vi "Sensor Read.vi"   [LabVIEW 2016]
uses:
  Drive/Drive Globals.vi
  Rotation/Rotation Globals.vi
types:
  T1 = typedef "CTRE_PigeonIMU_DeviceRef.ctl" = cluster{"DeviceStatus":errorcluster, "Device Number":u8, "Type":T2, "Device ID":u32}
  T2 = typedef "CTRE_PigeonIMU_ConnectionType.ctl" = u32
  T3 = typedef "CTRE_PigeonIMU_GlobalStatus.ctl" = cluster{"PigeonState":T4, "FusedHeading":cluster{"Heading":dbl, "Valid?":bool, "Fusing?":bool}, "YPR":cluster{"Yaw":dbl, "Pitch":dbl, "Roll":dbl}, "Compass":cluster{"Heading":dbl, "Magnitude":dbl, "Absolute Heading":dbl}, "Accelerometer":cluster{"Biased":cluster{"X":i16, "Y":i16, "Z":i16, "Norm":i16}, "Angles":cluster{"XZ Tilt":dbl, "YZ Tilt":dbl, "XY Tilt":dbl}}, "Magnetometer":cluster{"Raw":cluster{"X":i16, "Y":i16, "Z":i16}, "Biased":cluster{"X":i16, "Y":i16, "Z":i16}}, "Gyro":cluster{"X":dbl, "Y":dbl, "Z":dbl, "Norm":dbl}, "6D Quaternian":cluster{"W":dbl, "X":dbl, "Y":dbl, "Z":dbl}, "Temp. (C)":dbl, "UpTime":u32, "StartupStatus":cluster{"ResetCount":i32, "ResetFlags":i32, "FirmwareVersion":i32, "HasReset?":bool}, "Calibration":cluster{"CurrentMode":T5, "LastCalError":i32, "CalBooting?":bool}, "CAN Error":errorcluster, "AccumGyro":cluster{"X":dbl, "Y":dbl, "Z":dbl}, "Usage Frame":u32}
  T4 = typedef "CTRE_PigeonIMU_PigeonState.ctl" = enum16{"NoComm", "Initializing", "Ready", "UserCalibration"}
  T5 = typedef "CTRE_PigeonIMU_CalibrationMode.ctl" = u16
  T6 = typedef "WPI_SwitchDevRef.ctl" = cluster{"DevStatus":errorcluster, "DIO Channel":T7, "CntIndex":T8, "Normally Closed":bool}
  T7 = typedef "FPGA_DIOChannel.ctl" = enum8{"DIO 0", "DIO 1", "DIO 2", "DIO 3", "DIO 4", "DIO 5", "DIO 6", "DIO 7", "DIO 8", "DIO 9", "DIO MXP 0", "DIO MXP 1", "DIO MXP 2", "DIO MXP 3", "DIO MXP 4", "DIO MXP 5", "DIO MXP 6", "DIO MXP 7", "DIO MXP 8", "DIO MXP 9", "DIO MXP 10", "DIO MXP 11", "DIO MXP 12", "DIO MXP 13", "DIO MXP 14", "DIO MXP 15", "SPI Port CS1", "SPI Port CS2", "SPI Port CS3", "SPI Port MISO", "SPI Port MOSI", "Invalid"}
  T8 = typedef "FPGA_CounterCtrSystemIndex.ctl" = enum8{"Ctr 0", "Ctr 1", "Ctr 2", "Ctr 3", "Ctr 4", "Ctr 5", "Ctr 6", "Ctr 7", "Invalid"}
  T9 = typedef "WPI_EncoderDevRef.ctl" = cluster{"DevStatus":errorcluster, "EncoderIndex":T10, "CounterIndex":T8, "DistancePerCount":dbl, "Decoding Type":T11}
  T10 = typedef "FPGA_EncoderIdx.ctl" = enum8{"Enc 0", "Enc 1", "Enc 2", "Enc 3", "Enc 4", "Enc 5", "Enc 6", "Enc 7", "Invalid"}
  T11 = typedef "WPI_EncoderType.ctl" = enum16{"1x", "2x", "4x"}
  T12 = typedef "WPI_MotorControlDeviceRef.ctl" = cluster{"DeviceStatus":errorcluster, "Type":T13, "PWM":cluster{"PWM Channel":T14, "DeadBand":T15}, "CAN":cluster{"Device Number":u8, "SetOutput VI Ref":variant, "GetOutput VI Ref":variant, "Enable VI Ref":variant, "Disable VI Ref":variant, "Data":variant}, "Invert":bool}
  T13 = typedef "WPI_MotorControlType.ctl" = enum16{"PWM", "CAN"}
  T14 = typedef "FPGA_DIOPWMChannel.ctl" = enum8{"PWM 0", "PWM 1", "PWM 2", "PWM 3", "PWM 4", "PWM 5", "PWM 6", "PWM 7", "PWM 8", "PWM 9", "PWM MXP 0", "PWM MXP 1", "PWM MXP 2", "PWM MXP 3", "PWM MXP 4", "PWM MXP 5", "PWM MXP 6", "PWM MXP 7", "PWM MXP 8", "PWM MXP 9", "Invalid"}
  T15 = typedef "WPI_PWMDeadband.ctl" = cluster{"Name":string, "maxPositivePwm":i32, "minPositivePwm":i32, "centerPwm":i32, "maxNegativePwm":i32, "minNegativePwm":i32, "angularRange":u16}
  T16 = typedef "WPI_CANTalonSRX_GlobalStatus.ctl" = cluster{"Applied Throttle":dbl, "Module Enabled":bool, "CAN Error":errorcluster, "Closed Loop Error":dbl, "Forward Limit Switch Closed":bool, "Reverse Limit Switch Closed":bool, "Sensor Position":dbl, "Sensor Velocity":dbl, "Current":dbl, "Sticky Fault - Over Temp":bool, "Sticky Fault - Under Voltage":bool, "Sticky Fault - Forward Limit":bool, "Sticky Fault - Reverse Limit":bool, "Sticky Fault - Forward Soft Limit":bool, "Sticky Fault - Reverse Soft Limit":bool, "Brake is Enabled":bool, "Encoder Position":dbl, "Encoder Velocity":dbl, "Encoder Index Count":dbl, "Encoder A Pin State":bool, "Encoder B Pin State":bool, "Encoder Index Pin State":bool, "Analog In":dbl, "Analog In Velocity":dbl, "Temperature (C)":dbl, "Battery Voltage":dbl, "Control 5 Is Supported":bool, "Current Profile Slot Select":dbl, "Pos Div 8":bool, "Vel Div 4":bool, "Pulse Width Position":i32, "Pulse Width Velocity":i32, "Pulse Width Rise To Rise (us)":i32, "Pulse Width Rise To Fall (us)":i32, "Mot Prof Active Is Under Run":bool, "Mot Prof Active Has Under Run":bool, "Mot Prof Active Is Last":bool, "Mot Prof Active Velocity Only":bool, "Mot Prof Active Is Valid":bool, "Mot Prof Buffer Is Full":bool, "Mot Prof Active Profile Slot Select":i32, "Mot Prof NextID":i32, "Mot Prof Count":i32, "Mot Prof Active Velocity":dbl, "Mot Prof Active Position":dbl, "Mot Prof Output Enable":i32, "UsageFrame":u32, "Motion Magic Active Trajectory":cluster{"Velocity":dbl, "Position":dbl}}
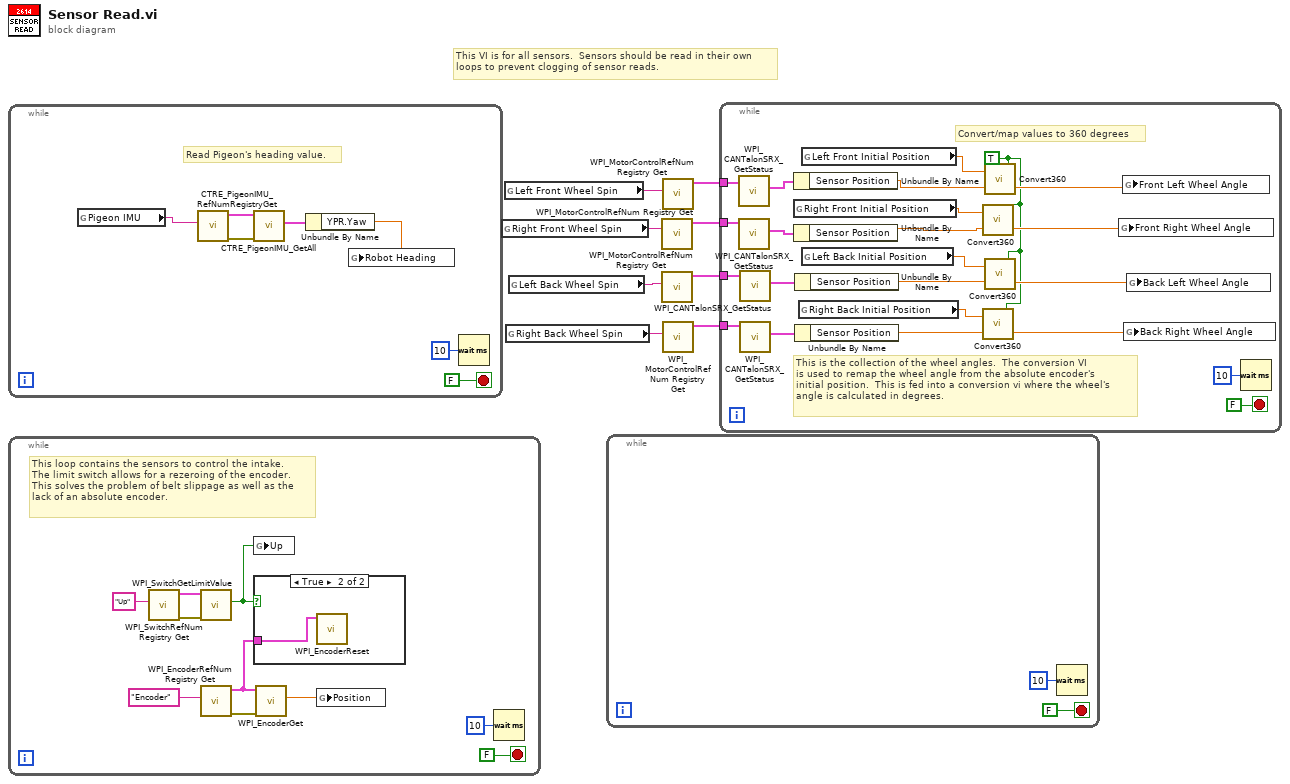
[diagram p0: block diagram]
diagram:
  # "This VI is for all sensors.  Sensors should be read in their own \nloops to prevent clogging of sensor reads."
  n1 = while {
    stop <- FALSE stop-if-true
    # "Read Pigeon's heading value."
    n2 = global read "Drive Globals.vi" "Pigeon IMU"() -> (w13:string)
    n3 = call <vilib>:"CTRE_PigeonIMU_RefNumRegistryGet.vi"("refnum name"=w13) -> ("error out"=w12:errorcluster, "PigeonIMUDevRef"=w11:T1)  [unwired: 9 in]
    n4 = call <vilib>:"CTRE_PigeonIMU_GetAll.vi"("error in (no error)"=w12, "PigeonIMUDevRef"=w11) -> ("Get All"=w10:T3)  [unwired: 7 in, 2 out]
    n5 = Unbundle By Name(w10) -> ("YPR.Yaw"=w9:dbl)
    n6 = global write "Drive Globals.vi" "Robot Heading"(w9) -> ()
    n7 = Wait (ms)(milliseconds to wait=u32 10) -> ()  [unwired: 1 out]
  }
  n8 = while {
    stop <- FALSE stop-if-true
    # "This loop contains the sensors to control the intake. \nThe limit switch allows for a rezeroing of the encoder.\nThis solves the problem of belt slippage as well as the\nlack of an absolute encoder."
    n9 = call <vilib>:"WPI_SwitchRefNum Registry Get.vi"("refnum name"="Up") -> ("error out"=w20:errorcluster, "SwitchDevRef"=w19:T6)  [unwired: 9 in]
    n10 = call <vilib>:"WPI_SwitchGetLimitValue.vi"("error in (no error)"=w20, "SwitchDevRef"=w19) -> ("Switch Pressed"=w17:bool)  [unwired: 7 in, 2 out]
    n11 = call <vilib>:"WPI_EncoderRefNum Registry Get.vi"("refnum name"="Encoder") -> ("error out"=w22:errorcluster, "EncoderDevRef"=w16:T9)  [unwired: 9 in]
    n12 = global write "Rotation Globals.vi" "Up"(w17) -> ()
    n13 = case shown="True" w17 {
      tunnel: w16 -> [_ w26]
      frame False {
      }
      frame True {
        n14 = call <vilib>:"WPI_EncoderReset.vi"("EncoderDevRef"=w26) -> ()  [unwired: 9 in, 2 out]
      }
    }
    n15 = call <vilib>:"WPI_EncoderGet.vi"("error in (no error)"=w22, "EncoderDevRef"=w16) -> ("Distance"=w21:dbl)  [unwired: 4 in, 5 out]
    n16 = global write "Rotation Globals.vi" "Position"(w21) -> ()
    n17 = Wait (ms)(milliseconds to wait=u32 10) -> ()  [unwired: 1 out]
  }
  n18 = global read "Drive Globals.vi" "Right Front Wheel Spin"() -> (w3:string)
  n19 = global read "Drive Globals.vi" "Left Front Wheel Spin"() -> (w4:string)
  n20 = global read "Drive Globals.vi" "Right Back Wheel Spin"() -> (w2:string)
  n21 = global read "Drive Globals.vi" "Left Back Wheel Spin"() -> (w1:string)
  n22 = while {
    stop <- FALSE stop-if-true
    n23 = Wait (ms)(milliseconds to wait=u32 10) -> ()  [unwired: 1 out]
  }
  n24 = call <vilib>:"WPI_MotorControlRefNum Registry Get.vi"("refnum name"=w3) -> ("MotorControlDevRef"=w6:T12)  [unwired: 9 in, 1 out]
  n25 = call <vilib>:"WPI_MotorControlRefNum Registry Get.vi"("refnum name"=w1) -> ("MotorControlDevRef"=w7:T12)  [unwired: 9 in, 1 out]
  n26 = call <vilib>:"WPI_MotorControlRefNum Registry Get.vi"("refnum name"=w4) -> ("MotorControlDevRef"=w5:T12)  [unwired: 9 in, 1 out]
  n27 = call <vilib>:"WPI_MotorControlRefNum Registry Get.vi"("refnum name"=w2) -> ("MotorControlDevRef"=w8:T12)  [unwired: 9 in, 1 out]
  n28 = while {
    tunnel: w8 -> [w45]
    tunnel: w7 -> [w44]
    tunnel: w6 -> [w43]
    tunnel: w5 -> [w42]
    stop <- FALSE stop-if-true
    w34 = TRUE ("Reverse")
    # "This is the collection of the wheel angles.  The conversion VI \nis used to remap the wheel angle from the absolute encoder's\ninitial position.  This is fed into a conversion vi where the wheel's\nangle is calculated in degrees."
    # "Convert/map values to 360 degrees"
    n29 = call <vilib>:"WPI_CANTalonSRX_GetStatus.vi"("CAN Talon SRX Ref"=w42) -> ("Talon SRX Status"=w49:T16)  [unwired: 8 in, 2 out]
    n30 = call <vilib>:"WPI_CANTalonSRX_GetStatus.vi"("CAN Talon SRX Ref"=w43) -> ("Talon SRX Status"=w48:T16)  [unwired: 8 in, 2 out]
    n31 = call <vilib>:"WPI_CANTalonSRX_GetStatus.vi"("CAN Talon SRX Ref"=w44) -> ("Talon SRX Status"=w47:T16)  [unwired: 8 in, 2 out]
    n32 = call <vilib>:"WPI_CANTalonSRX_GetStatus.vi"("CAN Talon SRX Ref"=w45) -> ("Talon SRX Status"=w46:T16)  [unwired: 8 in, 2 out]
    n33 = Unbundle By Name(w49) -> ("Sensor Position"=w35:dbl)
    n34 = global read "Drive Globals.vi" "Right Front Initial Position"() -> (w30:dbl)
    n35 = Unbundle By Name(w48) -> ("Sensor Position"=w37:dbl)
    n36 = Unbundle By Name(w47) -> ("Sensor Position"=w33:dbl)
    n37 = Unbundle By Name(w46) -> ("Sensor Position"=w41:dbl)
    n38 = global read "Drive Globals.vi" "Right Back Initial Position"() -> (w32:dbl)
    n39 = global read "Drive Globals.vi" "Left Front Initial Position"() -> (w29:dbl)
    n40 = global read "Drive Globals.vi" "Left Back Initial Position"() -> (w31:dbl)
    n41 = call "Convert360.vi"("Reverse"=w34, "Current Position"=w37, "Zero Position"=w30) -> ("Angle"=w38:dbl)
    n42 = call "Convert360.vi"("Reverse"=w34, "Current Position"=w41, "Zero Position"=w32) -> ("Angle"=w40:dbl)
    n43 = call "Convert360.vi"("Reverse"=w34, "Current Position"=w35, "Zero Position"=w29) -> ("Angle"=w36:dbl)
    n44 = call "Convert360.vi"("Reverse"=w34, "Current Position"=w33, "Zero Position"=w31) -> ("Angle"=w39:dbl)
    n45 = global write "Drive Globals.vi" "Front Right Wheel Angle"(w38) -> ()
    n46 = global write "Drive Globals.vi" "Front Left Wheel Angle"(w36) -> ()
    n47 = global write "Drive Globals.vi" "Back Right Wheel Angle"(w40) -> ()
    n48 = global write "Drive Globals.vi" "Back Left Wheel Angle"(w39) -> ()
    n49 = Wait (ms)(milliseconds to wait=u32 10) -> ()  [unwired: 1 out]
  }
